vi "main.vi"() -> ()   [LabVIEW 2015]
uses:
  Controls/state.ctl
  Controls/File action.ctl
  Controls/Message.ctl
  Controls/Users data.ctl
  Controls/user.ctl
  Controls/Get-Set.ctl
  Controls/Approved order.ctl
  Controls/Account action.ctl
panel:
  out "error out":errorcluster
  in  "error in":errorcluster
  in  "Enter":bool
  in  "User Input":string
  in  "Right Buttons":T1
  out "Right Menu":T2
  in  "Left Buttons":T1
  out "Left Menu":T2
  in  "Card Simulator":bool
  out "ATM Messages":string
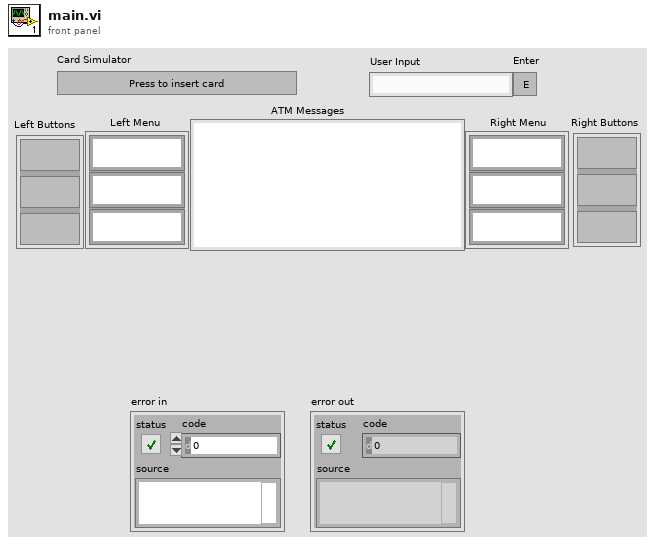
[diagram p1: front panel]
types:
  T1 = cluster{"Func Button":bool, "Func Button 2":bool, "Func Button 3":bool}
  T2 = cluster{"RFS String":string, "RFS String 2":string, "RFS String 3":string}
  T3 = typedef "File action.ctl" = enum16{"Read", "Write"}
  T4 = typedef "state.ctl" = enum16{"Run", "Error", "Exit", "Initialize"}
  T5 = typedef "Message.ctl" = enum16{"Session Terminate ", "Account Verification Failed", "Main Menu ", "Balance Inquiry", "Withdrawal Failed", "Withdrawal Complete", "Withdrawal", "Deposit Complete", "Deposit ", "Welcome "}
  T6 = enum8{"Enabled", "Disabled", "Disabled and Grayed Out"}
  T7 = typedef "Approved order.ctl" = enum16{"Withdraw", "Balance", "Deposit", "Verify"}
  T8 = typedef "Get-Set.ctl" = enum16{"Set", "Get"}
  T9 = typedef "Account action.ctl" = enum16{"Withdrawal", "Balance", "Deposit", "Validation"}
  T10 = typedef "Users data.ctl" = cluster{"Users":T11[], "Selected user id":i32}
  T11 = typedef "user.ctl" = cluster{"Code":string, "Full Name":string, "Money":string}
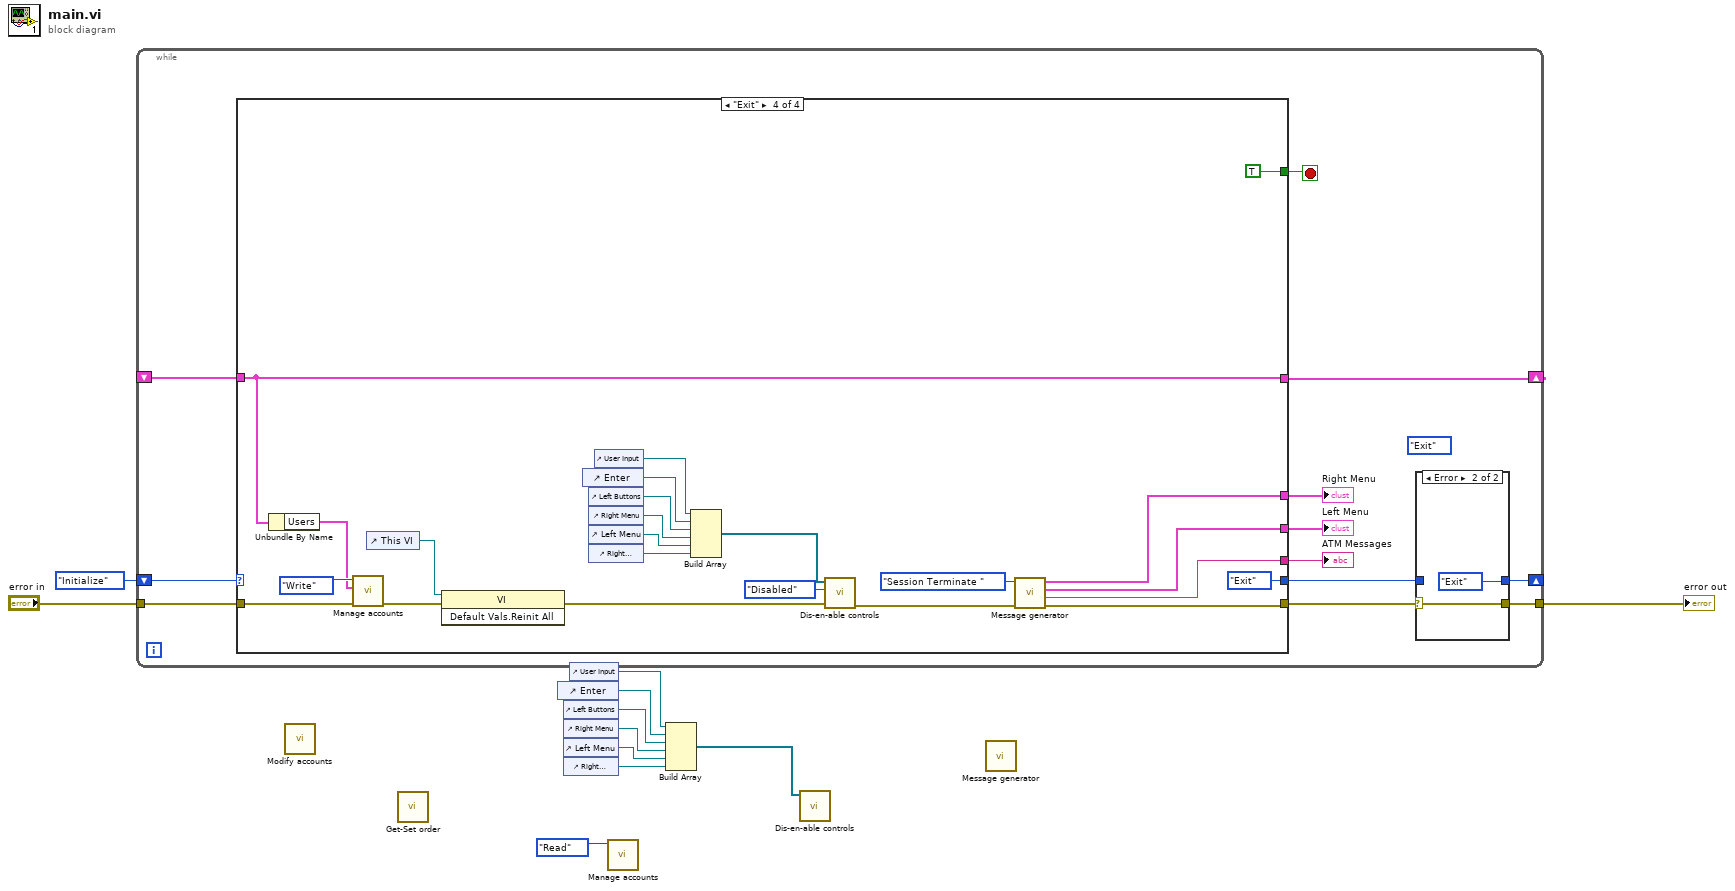
[diagram p0: block diagram]
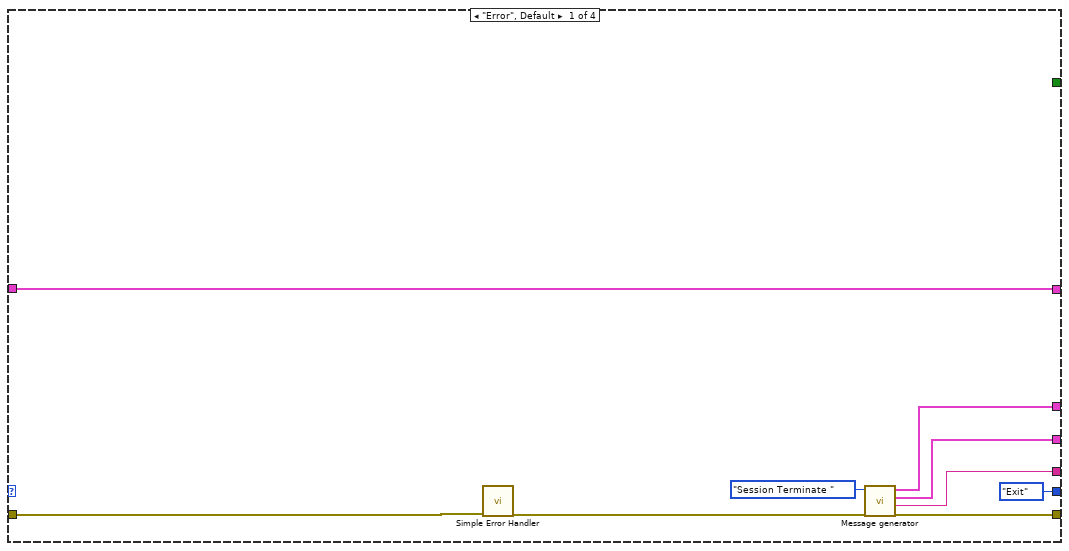
[diagram p3: hidden frame]
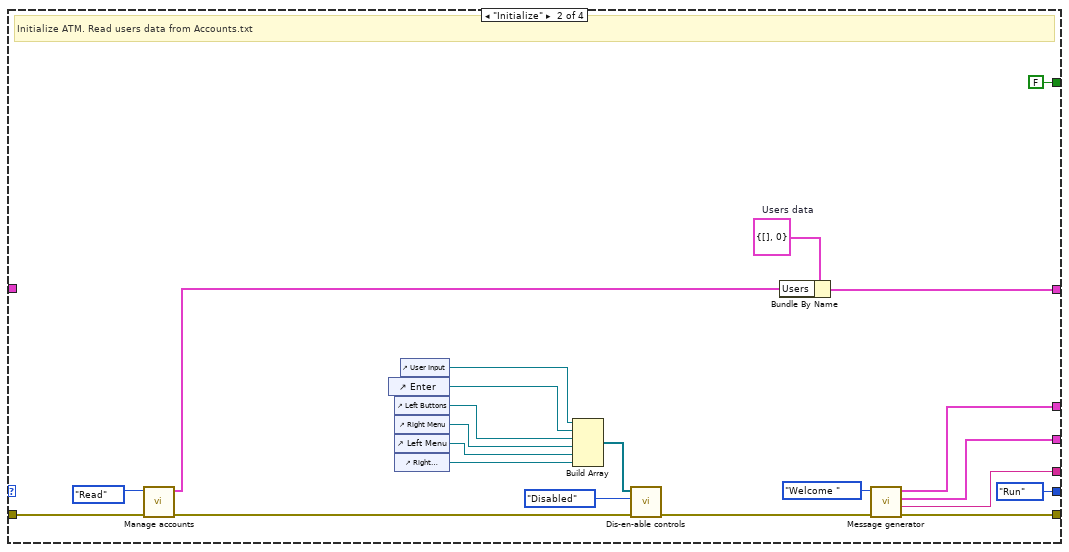
[diagram p4: hidden frame]
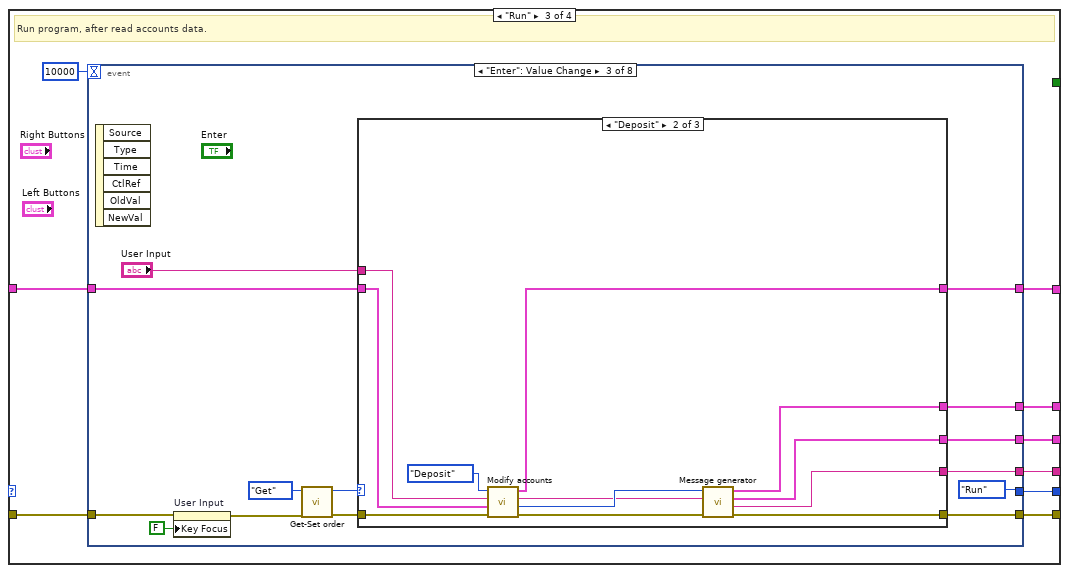
[diagram p5: hidden frame]
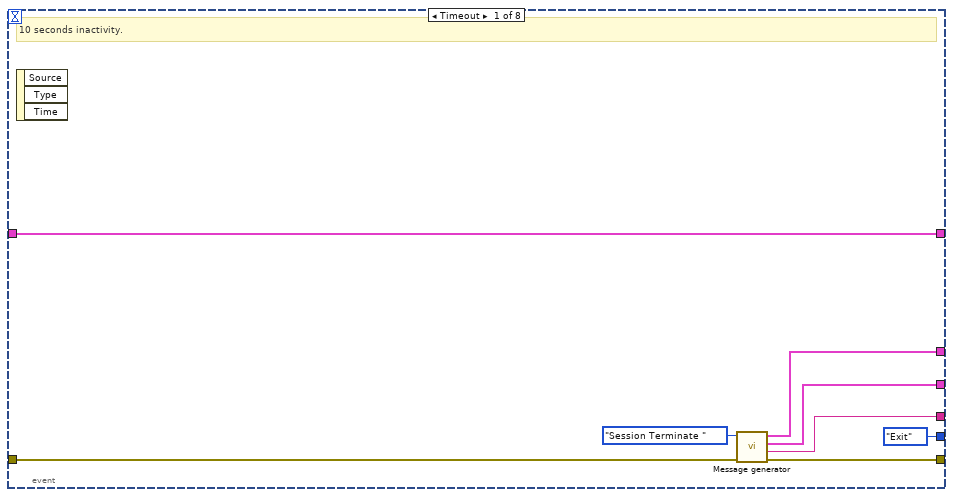
[diagram p6: hidden frame]
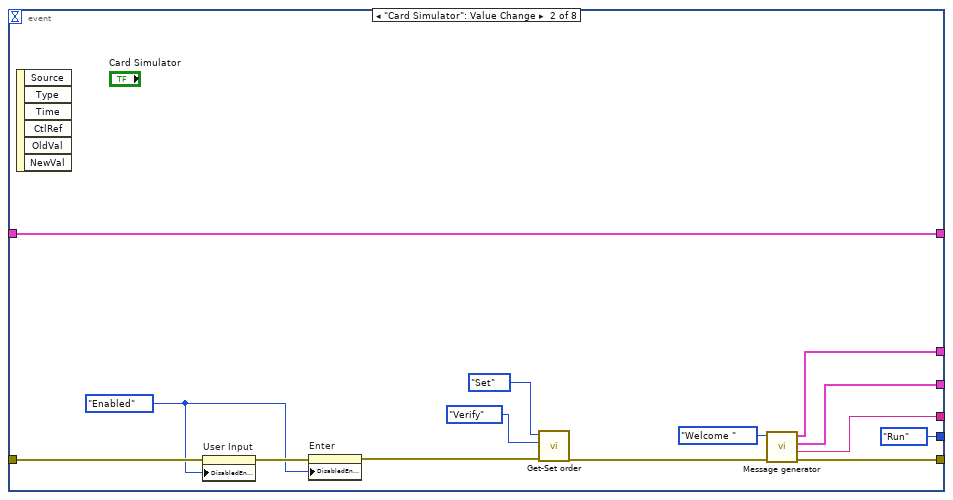
[diagram p7: hidden frame]
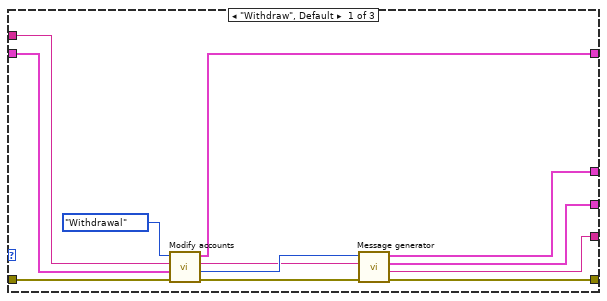
[diagram p8: hidden frame]
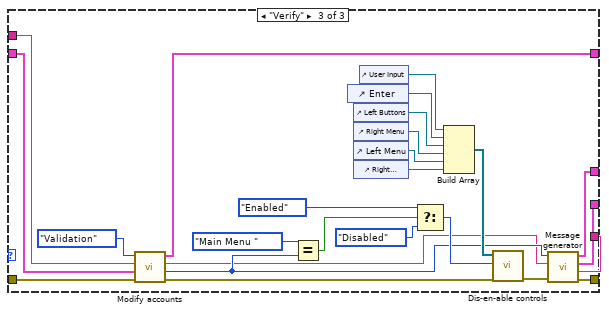
[diagram p9: hidden frame]
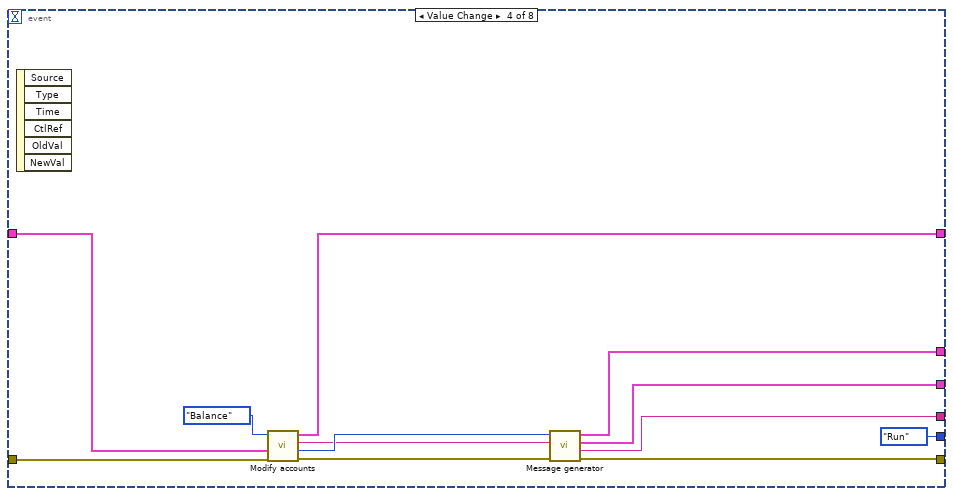
[diagram p10: hidden frame]
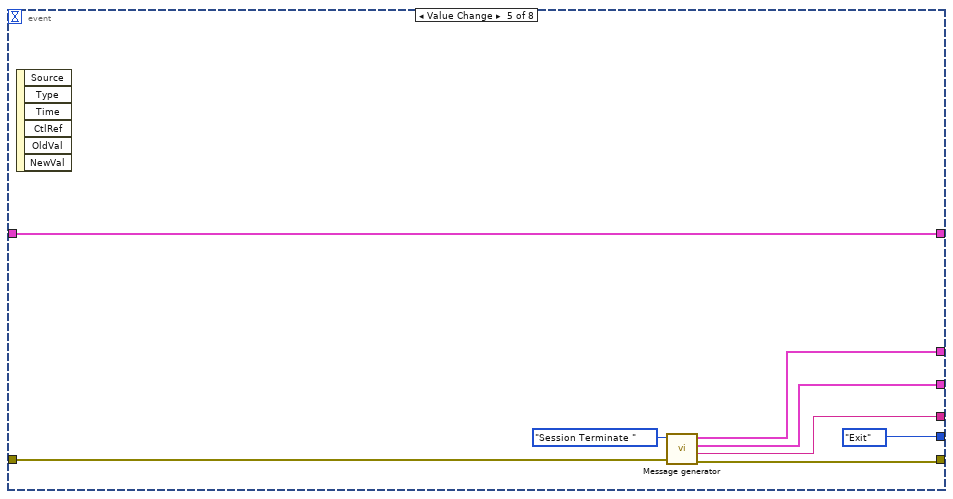
[diagram p11: hidden frame]
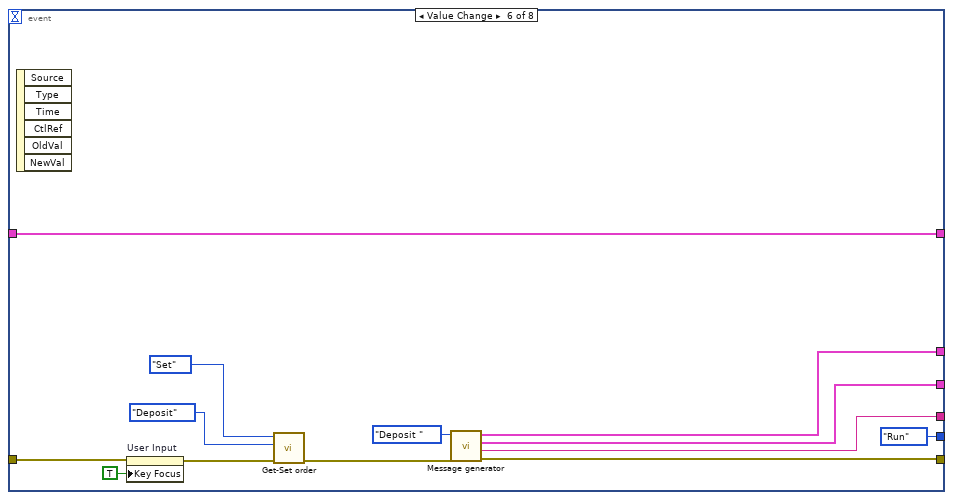
[diagram p12: hidden frame]
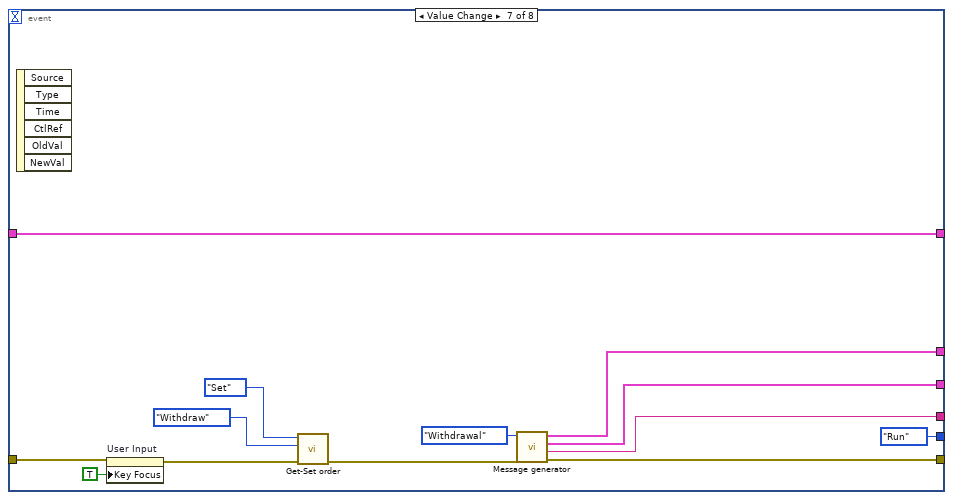
[diagram p13: hidden frame]
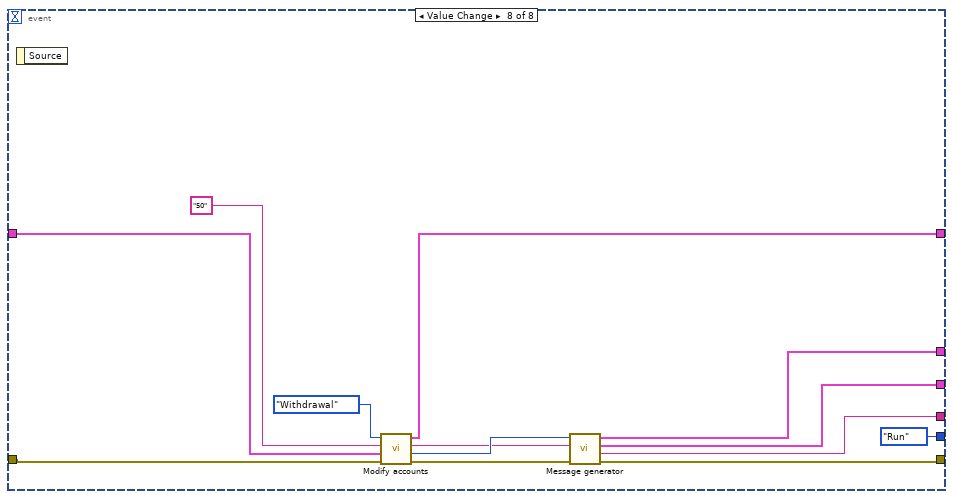
[diagram p14: hidden frame]
diagram:
  n1 = while {
    shift-right: [w12] -> _
    shift-left: state."Initialize" ("state") -> [w23]
    tunnel: "error in" -> [w22]
    tunnel: [w14] -> w9
    shift-right: [w21] -> _
    shift-left: _ -> [w17]
    stop <- w16 stop-if-true
    (unwired) state."Exit" ("state")
    n2 = case shown="\"Exit\"" w23 {
      tunnel: w22 -> [w36 w58 w66 w217]
      tunnel: [w35 w43 w65 w223] -> w15
      tunnel: [w29 w54 w61 w216] -> w21
      tunnel: [w32 w41 w64 w220] -> w20
      tunnel: [w31 w40 w63 w221] -> w19
      tunnel: [w30 w39 w62 w222] -> w18
      tunnel: w17 -> [w29 _ w60 w216]
      tunnel: [state."Exit" ("state") state."Run" ("state") w59 state."Exit" ("state")] -> w13
      tunnel: [_ FALSE _ TRUE] -> w16
      frame "Error", Default {
        n3 = call <vilib>:"Simple Error Handler.vi"("error in (no error)"=w36) -> ("error out"=w28:errorcluster)  [unwired: 4 in, 4 out]
        n4 = call "Message generator.vi"("error in"=w28, "Message"=Message."Session Terminate ") -> ("error out"=w35:errorcluster, "ATM Message"=w30:string, "Left Menu"=w31:T2, "Right Menu"=w32:T2)  [unwired: 6 in]
      }
      frame "Initialize" {
        w56 = T10 {"Users"=[], "Selected user id"=0}  # Users data
        # "Initialize ATM. Read users data from Accounts.txt"
        n5 = call "Manage accounts.vi"("error in"=w58, "File action"=File_action."Read") -> ("error out"=w46:errorcluster, "Users"=w55:T11[])  [unwired: 8 in]
        n6 = control-ref of="Enter"() -> (w48:refnum<vi>)
        n7 = control-ref of="Left Buttons"() -> (w49:refnum<vi>)
        n8 = control-ref of="Right Menu"() -> (w50:refnum<vi>)
        n9 = control-ref of="Left Menu"() -> (w51:refnum<vi>)
        n10 = control-ref of="Right Buttons"() -> (w52:refnum<vi>)
        n11 = control-ref of="User Input"() -> (w47:refnum<vi>)
        n12 = Build Array(w47, w48, w49, w50, w51, w52) -> (w53:refnum<vi>[])
        n13 = call "Dis-en-able controls.vi"("error in (no error)"=w46, "State"=T6."Disabled", "Array"=w53) -> ("error out"=w44:errorcluster)  [unwired: 8 in]
        n14 = Bundle By Name(cluster=w56, "Users"=w55) -> (w54:T10)
        n15 = call "Message generator.vi"("error in"=w44, "Message"=Message."Welcome ") -> ("error out"=w43:errorcluster, "ATM Message"=w39:string, "Left Menu"=w40:T2, "Right Menu"=w41:T2)  [unwired: 6 in]
      }
      frame "Run" {
        # "Run program, after read accounts data."
        n16 = event shown="[2] \"Enter\": Value Change" {
          selector: _ -> [_ _ _ _ _ _ _ _]
          dyn-events: _ -> [_ _ _ _ _ _ _ _]
          timeout: 10000 -> [_ _ _ _ _ _ _ _]
          tunnel: w66 -> [w75 w89 w94 w160 w171 w185 w198 w207]
          tunnel: [w74 w87 w98 w159 w170 w182 w195 w206] -> w65
          tunnel: [w69 w84 w95 w154 w166 w178 w192 w202] -> w64
          tunnel: [w68 w83 w96 w155 w167 w179 w193 w203] -> w63
          tunnel: [w71 w82 w97 w156 w168 w180 w194 w204] -> w62
          tunnel: [w72 w81 w99 w157 w165 w177 w191 w200] -> w61
          tunnel: w60 -> [w72 w81 w100 w158 w165 w177 w191 w201]
          tunnel: [state."Exit" ("state") state."Run" ("state") state."Run" ("state") state."Run" ("state") state."Exit" ("state") state."Run" ("state") state."Run" ("state") state."Run" ("state")] -> w59
          event Timeout {
            # "10 seconds inactivity."
            n17 = event-data() -> ()  [unwired: 1 in, 3 out]
            n18 = call "Message generator.vi"("error in"=w75, "Message"=Message."Session Terminate ") -> ("error out"=w74:errorcluster, "ATM Message"=w71:string, "Left Menu"=w68:T2, "Right Menu"=w69:T2)  [unwired: 6 in]
          }
          event "Card Simulator": Value Change {
            w86 = T6."Enabled" ("Disabled")
            n19 = event-data() -> ()  [unwired: 1 in, 6 out]
            n20 = property on="User Input" class="Str"(error in=w89, "DisabledEnum"=w86) -> (error out=w88:errorcluster)  [unwired: 1 in, 1 out]
            n21 = property on="Enter" class="Bool"(error in=w88, "DisabledEnum"=w86) -> (error out=w80:errorcluster)  [unwired: 1 in, 1 out]
            n22 = call "Get-Set order.vi"("error in"=w80, "Approved order in"=Approved_order."Verify", "Get-Set"=Get-Set."Set") -> ("error out"=w79:errorcluster)  [unwired: 7 in, 1 out]
            n23 = call "Message generator.vi"("error in"=w79, "Message"=Message."Welcome ") -> ("error out"=w87:errorcluster, "ATM Message"=w82:string, "Left Menu"=w83:T2, "Right Menu"=w84:T2)  [unwired: 6 in]
          }
          event "Enter": Value Change {
            n24 = event-data() -> ()  [unwired: 1 in, 6 out]
            n25 = property on="User Input" class="Str"(error in=w94, "Key Focus"=FALSE) -> (error out=w93:errorcluster)  [unwired: 1 in, 1 out]
            n26 = call "Get-Set order.vi"("error in"=w93, "Get-Set"=Get-Set."Get") -> ("error out"=w103:errorcluster, "Approved order out"=w102:T7)  [unwired: 8 in]
            n27 = case shown="\"Deposit\"" w102 {
              tunnel: w103 -> [w115 w127 w152]
              tunnel: w100 -> [w114 w125 w150]
              tunnel: [w109 w121 w149] -> w99
              tunnel: [w110 w119 w132] -> w98
              tunnel: [w106 w118 w131] -> w97
              tunnel: [w105 w117 w130] -> w96
              tunnel: [w104 w116 w129] -> w95
              tunnel: "User Input" -> [w113 w126 w128]
              frame "Withdraw", Default {
                n28 = call "Modify accounts.vi"("error in"=w115, "Users data"=w114, "User input"=w113, "Account action"=Account_action."Withdrawal") -> ("error out"=w111:errorcluster, "Message"=w108:T5, "User input output"=w107:string, "Users data out"=w109:T10)  [unwired: 4 in]
                n29 = call "Message generator.vi"("error in"=w111, "Account info"=w107, "Message"=w108) -> ("error out"=w110:errorcluster, "ATM Message"=w106:string, "Left Menu"=w105:T2, "Right Menu"=w104:T2)  [unwired: 5 in]
              }
              frame "Deposit" {
                n30 = call "Modify accounts.vi"("error in"=w127, "Users data"=w125, "User input"=w126, "Account action"=Account_action."Deposit") -> ("error out"=w123:errorcluster, "Message"=w122:T5, "User input output"=w120:string, "Users data out"=w121:T10)  [unwired: 4 in]
                n31 = call "Message generator.vi"("error in"=w123, "Account info"=w120, "Message"=w122) -> ("error out"=w119:errorcluster, "ATM Message"=w118:string, "Left Menu"=w117:T2, "Right Menu"=w116:T2)  [unwired: 5 in]
              }
              frame "Verify" {
                n32 = call "Modify accounts.vi"("error in"=w152, "Users data"=w150, "User input"=w128, "Account action"=Account_action."Validation") -> ("error out"=w141:errorcluster, "Message"=w134:T5, "User input output"=w133:string, "Users data out"=w149:T10)  [unwired: 4 in]
                n33 = Equal?(x=Message."Main Menu ", y=w134) -> (x = y?=w138:bool)
                n34 = control-ref of="Enter"() -> (w143:refnum<vi>)
                n35 = control-ref of="Left Buttons"() -> (w144:refnum<vi>)
                n36 = control-ref of="Right Menu"() -> (w145:refnum<vi>)
                n37 = control-ref of="Left Menu"() -> (w146:refnum<vi>)
                n38 = control-ref of="Right Buttons"() -> (w147:refnum<vi>)
                n39 = control-ref of="User Input"() -> (w142:refnum<vi>)
                n40 = Select(t=T6."Enabled" ("State"), s=w138, f=T6."Disabled" ("State")) -> (s? t:f=w135:T6)
                n41 = Build Array(w142, w143, w144, w145, w146, w147) -> (w148:refnum<vi>[])
                n42 = call "Dis-en-able controls.vi"("error in (no error)"=w141, "State"=w135, "Array"=w148) -> ("error out"=w140:errorcluster)  [unwired: 8 in]
                n43 = call "Message generator.vi"("error in"=w140, "Account info"=w133, "Message"=w134) -> ("error out"=w132:errorcluster, "ATM Message"=w131:string, "Left Menu"=w130:T2, "Right Menu"=w129:T2)  [unwired: 5 in]
              }
            }
          }
          event "Left Buttons.Func Button 2": Value Change {
            n44 = event-data() -> ()  [unwired: 1 in, 6 out]
            n45 = call "Modify accounts.vi"("error in"=w160, "Users data"=w158, "Account action"=Account_action."Balance") -> ("error out"=w163:errorcluster, "Message"=w162:T5, "User input output"=w161:string, "Users data out"=w157:T10)  [unwired: 5 in]
            n46 = call "Message generator.vi"("error in"=w163, "Account info"=w161, "Message"=w162) -> ("error out"=w159:errorcluster, "ATM Message"=w156:string, "Left Menu"=w155:T2, "Right Menu"=w154:T2)  [unwired: 5 in]
          }
          event "Left Buttons.Func Button 3": Value Change {
            n47 = event-data() -> ()  [unwired: 1 in, 6 out]
            n48 = call "Message generator.vi"("error in"=w171, "Message"=Message."Session Terminate ") -> ("error out"=w170:errorcluster, "ATM Message"=w168:string, "Left Menu"=w167:T2, "Right Menu"=w166:T2)  [unwired: 6 in]
          }
          event "Right Buttons.Func Button": Value Change {
            n49 = event-data() -> ()  [unwired: 1 in, 6 out]
            n50 = property on="User Input" class="Str"(error in=w185, "Key Focus"=TRUE) -> (error out=w176:errorcluster)  [unwired: 1 in, 1 out]
            n51 = call "Get-Set order.vi"("error in"=w176, "Approved order in"=Approved_order."Deposit", "Get-Set"=Get-Set."Set") -> ("error out"=w175:errorcluster)  [unwired: 7 in, 1 out]
            n52 = call "Message generator.vi"("error in"=w175, "Message"=Message."Deposit ") -> ("error out"=w182:errorcluster, "ATM Message"=w180:string, "Left Menu"=w179:T2, "Right Menu"=w178:T2)  [unwired: 6 in]
          }
          event "Right Buttons.Func Button 2": Value Change {
            n53 = event-data() -> ()  [unwired: 1 in, 6 out]
            n54 = property on="User Input" class="Str"(error in=w198, "Key Focus"=TRUE) -> (error out=w189:errorcluster)  [unwired: 1 in, 1 out]
            n55 = call "Get-Set order.vi"("error in"=w189, "Approved order in"=Approved_order."Withdraw", "Get-Set"=Get-Set."Set") -> ("error out"=w188:errorcluster)  [unwired: 7 in, 1 out]
            n56 = call "Message generator.vi"("error in"=w188, "Message"=Message."Withdrawal") -> ("error out"=w195:errorcluster, "ATM Message"=w194:string, "Left Menu"=w193:T2, "Right Menu"=w192:T2)  [unwired: 6 in]
          }
          event "Right Buttons.Func Button 3": Value Change {
            n57 = event-data() -> ()  [unwired: 1 in, 1 out]
            n58 = call "Modify accounts.vi"("error in"=w207, "Users data"=w201, "User input"="50", "Account action"=Account_action."Withdrawal") -> ("error out"=w210:errorcluster, "Message"=w209:T5, "User input output"=w208:string, "Users data out"=w200:T10)  [unwired: 4 in]
            n59 = call "Message generator.vi"("error in"=w210, "Account info"=w208, "Message"=w209) -> ("error out"=w206:errorcluster, "ATM Message"=w204:string, "Left Menu"=w203:T2, "Right Menu"=w202:T2)  [unwired: 5 in]
          }
        }
      }
      frame "Exit" {
        n60 = Unbundle By Name(w216) -> ("Users"=w215:T11[])
        n61 = call "Manage accounts.vi"("error in"=w217, "Users"=w215, "File action"=File_action."Write") -> ("error out"=w214:errorcluster)  [unwired: 7 in, 1 out]
        n62 = control-ref of="This VI"() -> (w212:refnum<vi>)
        n63 = invoke class="VI" method="Default Vals.Reinit All"(reference=w212, error in=w214) -> (error out=w213:errorcluster)  [unwired: 1 in, 2 out]
        n64 = control-ref of="Enter"() -> (w229:refnum<vi>)
        n65 = control-ref of="Left Buttons"() -> (w230:refnum<vi>)
        n66 = control-ref of="Right Menu"() -> (w231:refnum<vi>)
        n67 = control-ref of="Left Menu"() -> (w232:refnum<vi>)
        n68 = control-ref of="Right Buttons"() -> (w233:refnum<vi>)
        n69 = control-ref of="User Input"() -> (w227:refnum<vi>)
        n70 = Build Array(w227, w229, w230, w231, w232, w233) -> (w234:refnum<vi>[])
        n71 = call "Dis-en-able controls.vi"("error in (no error)"=w213, "State"=T6."Disabled", "Array"=w234) -> ("error out"=w225:errorcluster)  [unwired: 8 in]
        n72 = call "Message generator.vi"("error in"=w225, "Message"=Message."Session Terminate ") -> ("error out"=w223:errorcluster, "ATM Message"=w222:string, "Left Menu"=w221:T2, "Right Menu"=w220:T2)  [unwired: 6 in]
      }
    }
    "ATM Messages" <- w18
    "Left Menu" <- w19
    "Right Menu" <- w20
    n73 = case shown="Error" w15 {
      selector: w15 -> [w25 w26]
      tunnel: [w25 w26] -> w14
      tunnel: w13 -> [w24 _]
      tunnel: [w24 state."Exit" ("state")] -> w12
      frame No Error {
      }
      frame Error {
      }
    }
  }
  "error out" <- w9
  n74 = call "Modify accounts.vi"() -> ()  [unwired: 8 in, 4 out]
  n75 = call "Get-Set order.vi"() -> ()  [unwired: 10 in, 2 out]
  n76 = control-ref of="Enter"() -> (w7:refnum<vi>)
  n77 = control-ref of="Left Buttons"() -> (w6:refnum<vi>)
  n78 = control-ref of="Right Menu"() -> (w5:refnum<vi>)
  n79 = control-ref of="Left Menu"() -> (w4:refnum<vi>)
  n80 = control-ref of="Right Buttons"() -> (w3:refnum<vi>)
  n81 = control-ref of="User Input"() -> (w8:refnum<vi>)
  n82 = call "Manage accounts.vi"("File action"=File_action."Read") -> ()  [unwired: 9 in, 2 out]
  n83 = Build Array(w8, w7, w6, w5, w4, w3) -> (w2:refnum<vi>[])
  n84 = call "Dis-en-able controls.vi"("Array"=w2) -> ()  [unwired: 10 in, 1 out]
  n85 = call "Message generator.vi"() -> ()  [unwired: 8 in, 4 out]
